vi "select_vector_waveforms.vi"(4 "Trace timestamp":timestamp, 6 "Decimated dt":dbl, 9 "Decimated trace":sgl[][][](array[numeric]), 10 "Reference":sgl[][](array[numeric]), 11 "Trace controls":T1[](array[typedef])) -> (3 "Waveforms out":waveform(sgl)[](array[waveform]))   [LabVIEW 2013]
uses:
  Trace controls.ctl
  probe_point.ctl
  <vilib>/Analysis/baseanly.llb/A x Vector.vi
  <vilib>/Analysis/NI_AALBase.lvlib
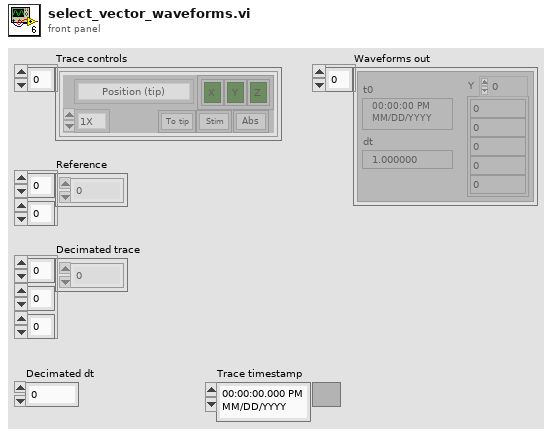
[diagram p1: front panel]
types:
  T1 = typedef "Trace controls.ctl" = cluster{"+ stim":bool, "Relative":bool, "Scale":enum16{"1X", "10X", "100X", "1KX", "10KX"}, "Probe point":T2, "XYZ selector":cluster{"Boolean":bool, "Boolean 2":bool, "Boolean 3":bool}, "To tip":bool}
  T2 = typedef "probe_point.ctl" = enum16{"Position (tip)", "Position (RCM)", "Null pos (tip)", "Null pos (RCM)", "V limiter (tip)", "V Limiter (RCM)", "Goal (tip)", "Goal (RCM)", "Link pos 0", "Link pos 1", "KF link pos 0", "KF link pos 1", "Link rate 0", "Link rate 1", "Link residue 0", "Link residue 1", "Link goal 0", "Link goal 1", "Rate limit 0", "Rate limit 1", "Link error 0", "Link error 1", "Controller 0", "Controller 1", "Output 0", "Output 1", "Drive 0", "Drive 1", "Stimulus 0", "Stimulus 1", "Trace data 0", "Trace data 1", "Analog data 0", "Analog data 1", "Status flags", "Light 0", "Light 1", "Light 2", "Light 3", "Light 4", "Light 5", "Goal origin", "Goal rotation 0", "Goal rotation 1", "Goal rotation 2", "Output origin", "Output rotation 0", "Output rotation 1", "Output rotation 2", "Handle origin", "Handle rotation 0", "Handle rotation 1", "Handle rotation 2", "Handle position", "Handle velocity", "Handle acceleration", "Handle angles", "Handle angle rates", "Handle pos residue", "Handle angle residue", "Trace length"}
  T3 = typedef "NI_Matrix.lvlib/RealMatrix.ctl" = dbl[][]
  T4 = cluster{"Boolean":bool, "Boolean 2":bool, "Boolean 3":bool}
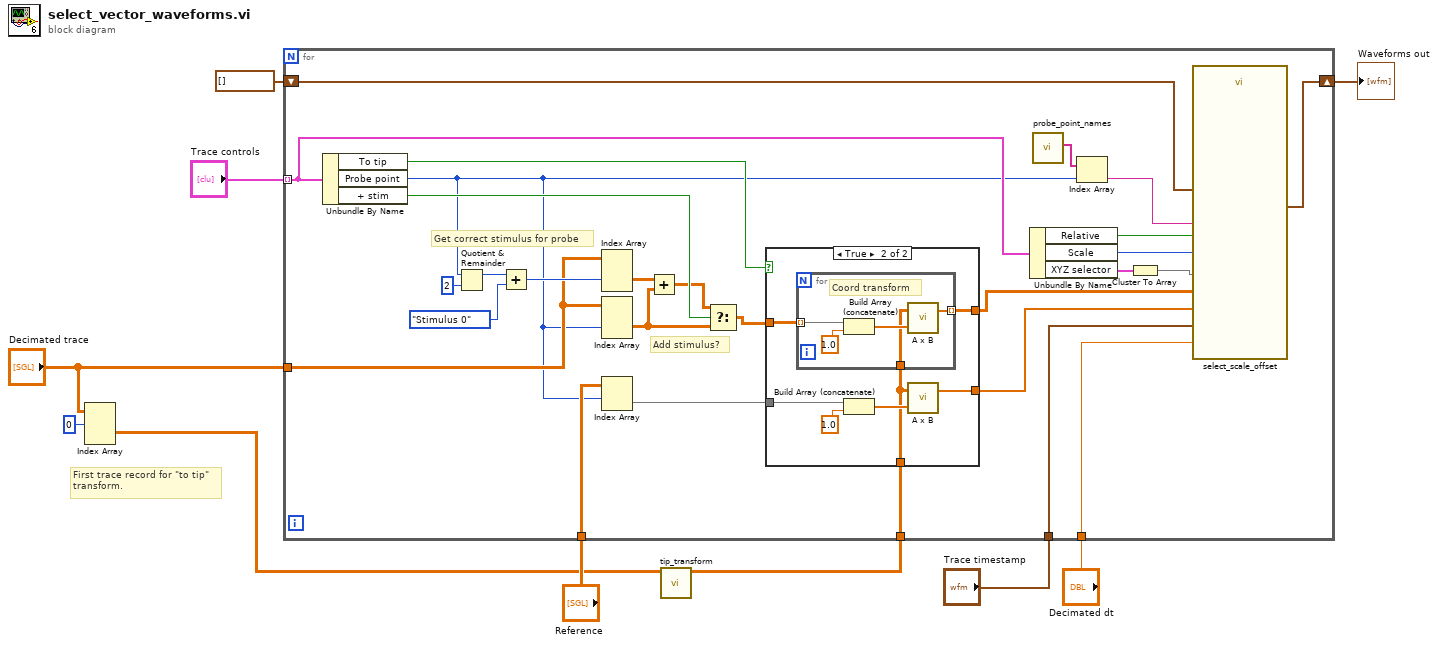
[diagram p0: block diagram]
diagram:
  # "First trace record for \"to tip\"\ntransform."
  n1 = Index Array(array="Decimated trace", index (dim 0)=0 ("index (page)")) -> (element=w1:sgl[][])  [unwired: 2 in]
  n2 = call "tip_transform.vi"("Trace record"=w1) -> ("To tip transform"=w5:T3)  [unwired: 10 in]
  n3 = for {
    shift-right: [w38] -> w8
    shift-left: waveform(sgl)[] [] -> [w21]
    tunnel: "Trace controls" -> [w22] mode=indexing
    tunnel: "Decimated dt" -> [w15]
    tunnel: w5 -> [w32]
    tunnel: "Decimated trace" -> [w27]
    tunnel: "Reference" -> [w24]
    tunnel: "Trace timestamp" -> [w11]
    # "Get correct stimulus for probe"
    # "Add stimulus?"
    n4 = Unbundle By Name(w22) -> ("To tip"=w25:bool, "Probe point"=w14:T2, "+ stim"=w36:bool)
    n5 = Quotient & Remainder(x=w14, y=2 ("index (page)")) -> (x-y*floor(x/y)=w28:i32)  [unwired: 1 out]
    n6 = Add(x=w28, y=probe_point."Stimulus 0" ("Probe point")) -> (x+y=w30:i32)
    n7 = Index Array(array=w27, index (dim 1)=w30) -> (element=w37:sgl[][])  [unwired: 2 in]
    n8 = Index Array(array=w27, index (dim 1)=w14) -> (element=w34:sgl[][])  [unwired: 2 in]
    n9 = Index Array(array=w24, index (row)=w14) -> (element=w13:sgl[])  [unwired: 1 in]
    n10 = Add(x=w37, y=w34) -> (x+y=w35:sgl[][])
    n11 = Select(t=w35, s=w36, f=w34) -> (s? t:f=w33:sgl[][])
    n12 = case shown="True" w25 {
      tunnel: w33 -> [w40 w47]
      tunnel: w32 -> [_ w44]
      tunnel: [w40 w46] -> w16
      tunnel: w13 -> [w39 w43]
      tunnel: [w39 w41] -> w12
      frame False {
        # "No coord transform"
      }
      frame True {
        n13 = for {
          tunnel: w47 -> [w51] mode=indexing
          tunnel: w44 -> [w48]
          tunnel: [w49] -> w46 mode=indexing
          # "Coord transform"
          n14 = Build Array (concatenate)(w51, sgl 1.0 ("Numeric")) -> (w50:sgl[])
          n15 = call-poly <vilib>:"A x B.vi"("Vector"=w50, "A"=w48) -> ("A x Vector"=w49:dbl[])  [unwired: 1 out]
        }
        n16 = Build Array (concatenate)(w43, sgl 1.0 ("Numeric")) -> (w45:sgl[])
        n17 = call-poly <vilib>:"A x B.vi"("Vector"=w45, "A"=w44) -> ("A x Vector"=w41:dbl[])  [unwired: 1 out]
      }
    }
    n18 = Unbundle By Name(w22) -> ("Relative"=w19:bool, "Scale"=w17:enum16{"1X", "10X", "100X", "1KX", "10KX"}, "XYZ selector"=w23:T4)
    n19 = call "probe_point_names.vi"() -> ("Names"=w26:string[])  [unwired: 11 in]
    n20 = Index Array(array=w26, index=w14) -> (element=w20:string)
    n21 = Cluster To Array(cluster=w23) -> (array=w18:bool[])
    n22 = call "select_scale_offset.vi"("Waveforms in"=w21, "Points"=w16, "Name"=w20, "Selector"=w18, "Scale"=w17, "Relative"=w19, "Decimated dt"=w15, "Trace timestamp"=w11, "Reference"=w12) -> ("Waveforms out"=w38:waveform(sgl)[])  [unwired: 6 in]
  }
  "Waveforms out" <- w8
